vi "Apply.vi"(8 "error in":errorcluster, 11 "AO DAQmx DC CFG in":refnum<class "AO DAQmx DC CFG.lvclass">) -> (0 "error out":errorcluster, 3 "AO DAQmx DC CFG out":refnum<class "AO DAQmx DC CFG.lvclass">)   [LabVIEW 2024, in "AO DAQmx DC CFG.lvclass"]
uses:
  AO DAQmx DC CFG.lvclass
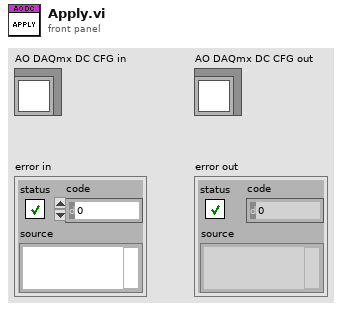
[diagram p1: front panel]
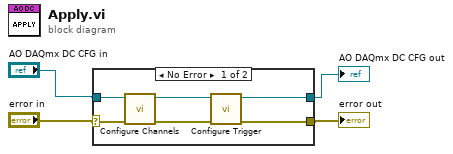
[diagram p0: block diagram]
diagram:
  n1 = case shown="No Error" "error in" {
    selector: "error in" -> [w9 w12]
    tunnel: "AO DAQmx DC CFG in" -> [w10 w11]
    tunnel: [w5 w12] -> w1
    tunnel: [w6 w11] -> w2
    frame No Error {
      n2 = call-dynamic "Configure Channels.vi"("error in"=w9, "AO DAQmx DC CFG in"=w10) -> ("error out"=w7:errorcluster, "AO DAQmx DC CFG out"=w8:refnum<class "AO DAQmx DC CFG.lvclass">)  [unwired: 8 in]
      n3 = call-dynamic "Configure Trigger.vi"("error in"=w7, "DAQmx Base CFG in"=w8) -> ("error out"=w5:errorcluster, "DAQmx Base CFG out"=w6:refnum<class "AO DAQmx DC CFG.lvclass">)  [unwired: 8 in]
    }
    frame Error {
    }
  }
  "error out" <- w1
  "AO DAQmx DC CFG out" <- w2
